vi "New Session SetUp.vi"(8 "error in (no error)":errorcluster, 10 "Stop Refnum":refnum<vi>, 11 "AMS TS3472 in":refnum<class "AMS TCS3472.lvclass">) -> (0 "error out":errorcluster, 3 "AMS TS3472 out":refnum<class "AMS TCS3472.lvclass">)   [LabVIEW 2016, in "AMS TS3472 Light Sensor.lvlib" / "AMS TCS3472.lvclass"]
uses:
  AMS TCS3472.lvclass
  Abstract Sensor/Abstract Sensor.lvclass
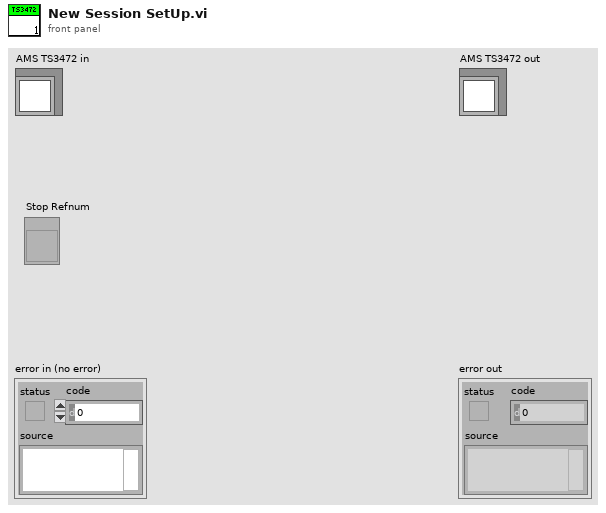
[diagram p1: front panel]
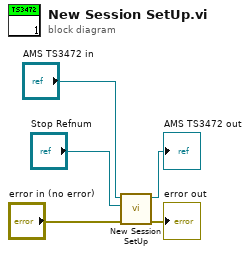
[diagram p0: block diagram]
diagram:
  n1 = call-parent "New Session SetUp.vi"("error in (no error)"="error in (no error)", "Stop Refnum"="Stop Refnum", "Abstract Sensor in"="AMS TS3472 in") -> ("error out"=→"error out":errorcluster, "Abstract Sensor out"=→"AMS TS3472 out":refnum<class "AMS TCS3472.lvclass">)  [unwired: 7 in]
